vi "Set Status Code.vi"(8 "error in (no error)":errorcluster, 10 "Status Code":u16, 11 "Response in":refnum<class "Response.lvclass">) -> (0 "error out":errorcluster, 3 "Response out":refnum<class "Response.lvclass">)   [LabVIEW 2020, in "HTTP Utils.lvlib" / "Response.lvclass"]
uses:
  Response.lvclass
  Response.lvclass/Response.ctl
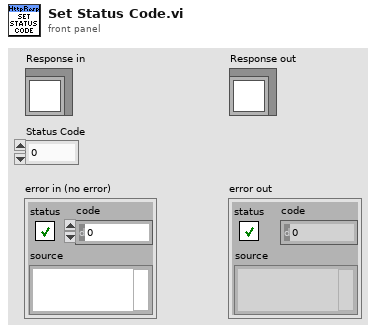
[diagram p1: front panel]
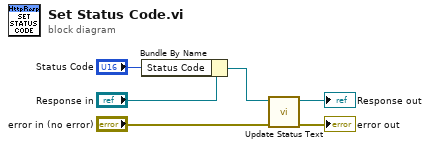
[diagram p0: block diagram]
diagram:
  n1 = Bundle By Name(cluster="Response in", "Status Code"="Status Code") -> (w3:refnum<class "Response.lvclass">)
  n2 = call "Update Status Text.vi"("error in (no error)"="error in (no error)", "Response in"=w3) -> ("error out"=→"error out":errorcluster, "Response out"=→"Response out":refnum<class "Response.lvclass">)  [unwired: 8 in]
